vi "VI Tree.vi"   [LabVIEW 2012, in "Phidget Magnetometer.lvlib"]
doc: "${Magnetometer:VITreeHeader}"
uses:
  <instrlib>/Phidgets/Phidget Magnetometer/Phidget Magnetometer.lvlib
  <instrlib>/Phidgets/Phidget Magnetometer/Public/MagnetometerStart.vi
  <instrlib>/Phidgets/Phidget Magnetometer/Public/MagnetometerOpen.vi
  <instrlib>/Phidgets/Phidget Magnetometer/Public/MagnetometerClose.vi
panel:
  # "(c) 2015 Phidgets Inc..  ALL RIGHTS RESERVED."
  # "SEE DIAGRAM\nFOR VI TREE."
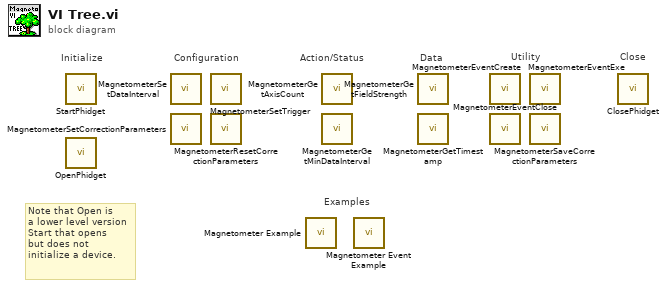
[diagram p0: block diagram]
diagram:
  # "Note that Open is\na lower level version\nStart that opens\nbut does not \ninitialize a device."
  # "Examples"
  # "Configuration"
  # "Utility"
  # "Data"
  # "Action/Status"
  # "Close"
  # "Initialize"
  n1 = call-poly <instrlib>:"StartPhidget.vi"() -> ()  [unwired: 12 in, 4 out]
  n2 = call-poly <instrlib>:"OpenPhidget.vi"() -> ()  [unwired: 8 in, 4 out]
  n3 = call <instrlib>:"MagnetometerSetDataInterval.vi"() -> ()  [unwired: 9 in, 2 out]
  n4 = call <instrlib>:"MagnetometerSetCorrectionParameters.vi"() -> ()  [unwired: 9 in, 2 out]
  n5 = call <instrlib>:"MagnetometerSetTrigger.vi"() -> ()  [unwired: 9 in, 2 out]
  n6 = call <instrlib>:"MagnetometerResetCorrectionParameters.vi"() -> ()  [unwired: 9 in, 2 out]
  n7 = call <instrlib>:"Magnetometer Example.vi"() -> ()  [unwired: 12 in]
  n8 = call <instrlib>:"MagnetometerGetAxisCount.vi"() -> ()  [unwired: 8 in, 3 out]
  n9 = call <instrlib>:"MagnetometerGetMinDataInterval.vi"() -> ()  [unwired: 8 in, 3 out]
  n10 = call <instrlib>:"Magnetometer Event Example.vi"() -> ()  [unwired: 12 in]
  n11 = call <instrlib>:"MagnetometerGetFieldStrength.vi"() -> ()  [unwired: 8 in, 3 out]
  n12 = call <instrlib>:"MagnetometerGetTimestamp.vi"() -> ()  [unwired: 8 in, 3 out]
  n13 = call <instrlib>:"MagnetometerEventCreate.vi"() -> ()  [unwired: 9 in, 3 out]
  n14 = call <instrlib>:"MagnetometerEventClose.vi"() -> ()  [unwired: 10 in, 2 out]
  n15 = call <instrlib>:"MagnetometerEventExe.vi"() -> ()  [unwired: 8 in, 8 out]
  n16 = call <instrlib>:"MagnetometerSaveCorrectionParameters.vi"() -> ()  [unwired: 9 in, 2 out]
  n17 = call-poly <instrlib>:"ClosePhidget.vi"() -> ()  [unwired: 11 in, 1 out]
